vi "0xE5 Записать все параметры типа int (SubVI).vi"(10 "Количество параметры типа int":i32, 11 "String in":string) -> (3 "String out":string)   [LabVIEW 2017, in "LV_Unicorn.lvlib"]
uses:
  LV_Unicorn.lvlib
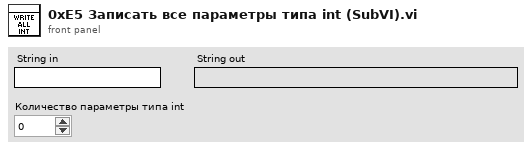
[diagram p1: front panel]
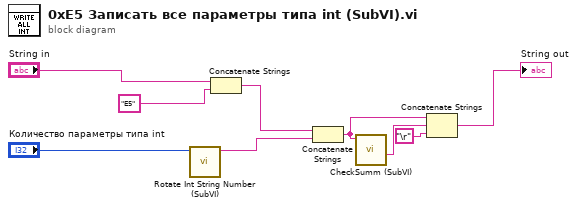
[diagram p0: block diagram]
diagram:
  n1 = call "Rotate Int String Number (SubVI).vi"("Int Number In"="Количество параметры типа int") -> ("Orig String"=w2:string)  [unwired: 8 in, 2 out]
  n2 = Concatenate Strings("String in", "E5" ("string")) -> (w7:string)
  n3 = Concatenate Strings(w7, w2) -> (w4:string)
  n4 = call "CheckSumm (SubVI).vi"("Input String"=w4) -> ("CheckSumm"=w3:string)  [unwired: 7 in, 3 out]
  n5 = Concatenate Strings(w4, w3, "\r") -> (→"String out":string)
